vi "N4_201_write_P.vi"(0 "DriverConnect in":T1={"InterfaceType"=enum."VISA", "OpenedSession"="", "InterfaceSettings"={"Interface"=enum."RS232", "EOS 4 read"=enum."LF (\\n)", "EOS 4 write"=enum."LF (\\n)", "TMO, ms"=10000, "Sett"=variant(cluster{"Baud Rate":u32, "Data Bits":u16, "Parity":u16, "Stop Bits":u16, "Flow Control":u16, "Eho":bool} {"Baud Rate"=75, "Data Bits"=0, "Parity"=0, "Stop Bits"=0, "Flow Control"=0, "Eho"=FALSE})}}, 1 "P":T8, 2 "RangeIsChanged?":T6=TRUE, 3 "Command Time (s)":T7=1.0, 11 "error in":T9, 12 "Error Code":T11, 14 "Driver Name":T10) -> (4 "DriverConnect out":T1={"InterfaceType"=enum."VISA", "OpenedSession"="", "InterfaceSettings"={"Interface"=enum."RS232", "EOS 4 read"=enum."LF (\\n)", "EOS 4 write"=enum."LF (\\n)", "TMO, ms"=10000, "Sett"=variant(cluster{"Baud Rate":u32, "Data Bits":u16, "Parity":u16, "Stop Bits":u16, "Flow Control":u16, "Eho":bool} {"Baud Rate"=75, "Data Bits"=0, "Parity"=0, "Stop Bits"=0, "Flow Control"=0, "Eho"=FALSE})}}, 15 "error out":T9)   [LabVIEW 2018]
uses:
  MOKO_LabViewLibrary/MokoLowLevel/MokoLowLovelControl/MLLC_ErrorCode.ctl
  MOKO_LabViewLibrary/MokoLowLevel/MokoLowLovelControl/MLLC_DriverName.ctl
  MOKO_LabViewLibrary/MokoLowLevel/MokoLowLovelControl/MLLC_Error.ctl
  MOKO_LabViewLibrary/MokoLowLevel/MokoLowLovelControl/MLLC_Command.ctl
  MOKO_LabViewLibrary/MokoLowLevel/MokoLowLovelControl/MLLC_Delay.ctl
  MOKO_LabViewLibrary/MokoLowLevel/MokoLowLovelControl/MLLC_Boolean.ctl
  MOKO_LabViewLibrary/MokoLowLevel/MokoLowLovelControl/MLLC_DriverConnectCluster.ctl
  MOKO_LabViewLibrary/MokoLowLevel/MokoLowLovelControl/MLLC_InterfaceType.ctl
  MOKO_LabViewLibrary/MokoLowLevel/MokoLowLovelControl/MLLC_OpenedSession.ctl
  MOKO_LabViewLibrary/MokoLowLevel/MokoLowLovelControl/MLLC_InterfaceSettings.ctl
  MOKO_LabViewLibrary/MokoLowLevel/MokoLowLovelControl/MLLC_InterfaceKind.ctl
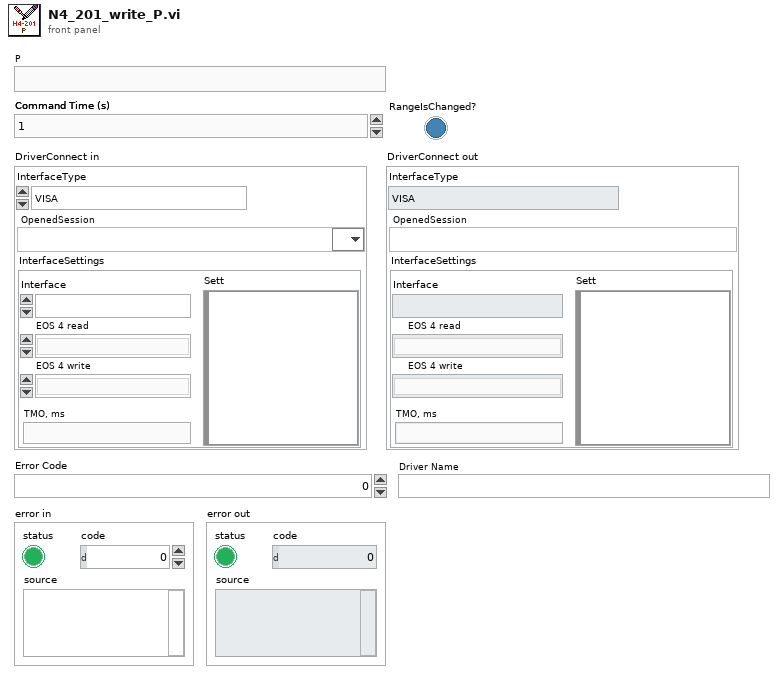
[diagram p1: front panel]
types:
  T1 = typedef "MLLC_DriverConnectCluster.ctl" = cluster{"InterfaceType":T2, "OpenedSession":T3, "InterfaceSettings":T4}
  T2 = typedef "MLLC_InterfaceType.ctl" = enum16{"VISA", "Prologix USB-GPIB"}
  T3 = typedef "MLLC_OpenedSession.ctl" = refnum<visa-resource-name>
  T4 = typedef "MLLC_InterfaceSettings.ctl" = cluster{"Interface":T5, "EOS 4 read":enum16{"Default (=EOS 4 write)", "CR (\\r)", "LF (\\n)", "None"}, "EOS 4 write":enum16{"CR+LF (\\r\\n)", "CR (\\r)", "LF (\\n)", "None"}, "TMO, ms":i32, "Sett":variant}
  T5 = typedef "MLLC_InterfaceKind.ctl" = enum16{"RS232", "GPIB", "USB", "Ethernet", "another"}
  T6 = typedef "MLLC_Boolean.ctl" = bool
  T7 = typedef "MLLC_Delay.ctl" = dbl
  T8 = typedef "MLLC_Command.ctl" = string
  T9 = typedef "MLLC_Error.ctl" = errorcluster
  T10 = typedef "MLLC_DriverName.ctl" = string
  T11 = typedef "MLLC_ErrorCode.ctl" = u32
  T12 = enum16{"Нет симуляции", "В ручную", "Игнорировать"}
  T13 = typedef "MLLC_Response.ctl" = string
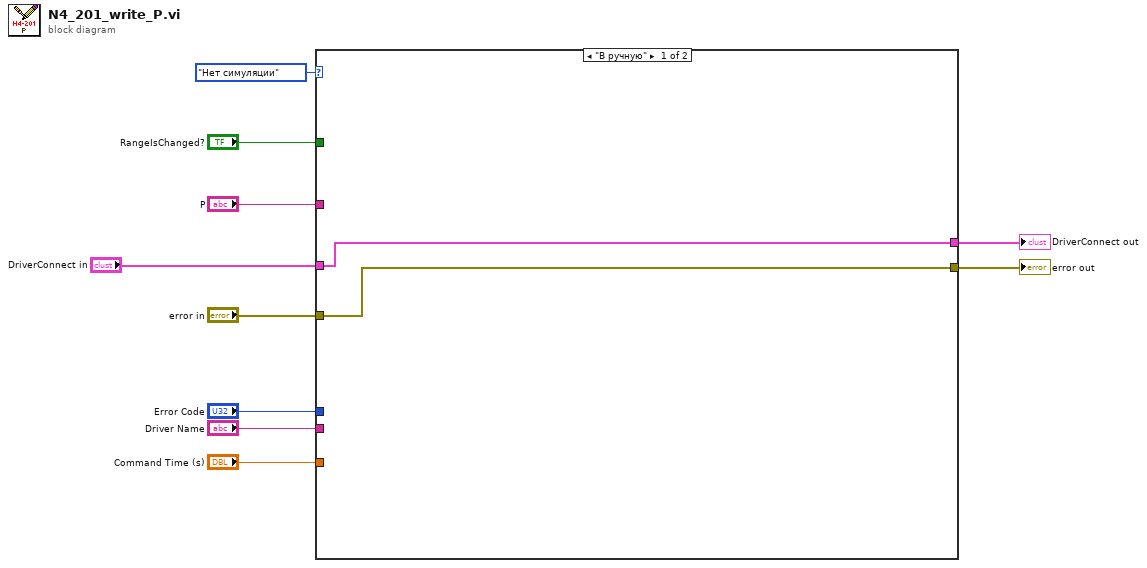
[diagram p0: block diagram]
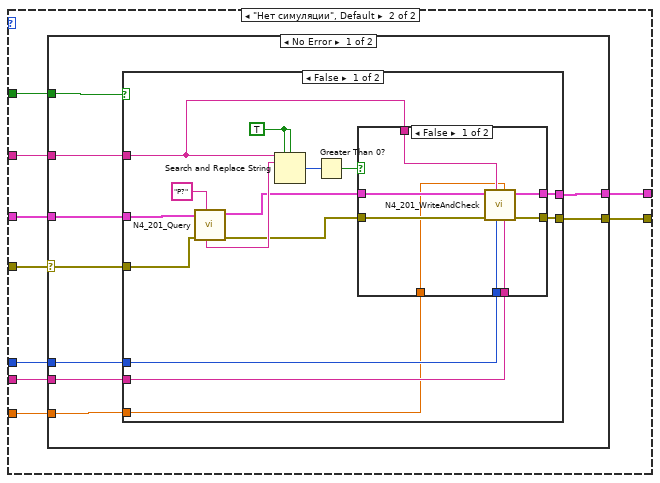
[diagram p2: hidden frame]
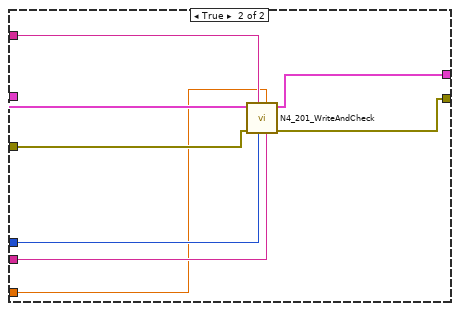
[diagram p4: hidden frame]
diagram:
  n1 = case shown="\"В ручную\"" T12."Нет симуляции" ("Simmulation") {
    tunnel: [w11 w21] -> w10
    tunnel: "Error Code" -> [_ w20]
    tunnel: "Driver Name" -> [_ w19]
    tunnel: "DriverConnect in" -> [w12 w18]
    tunnel: "error in" -> [w11 w17]
    tunnel: "P" -> [_ w16]
    tunnel: "Command Time (s)" -> [_ w15]
    tunnel: [w12 w14] -> w1
    tunnel: "RangeIsChanged?" -> [_ w13]
    frame "В ручную" {
    }
    frame "Нет симуляции", Default {
      n2 = case shown="No Error" w17 {
        selector: w17 -> [w25 w65]
        tunnel: [w27 w65] -> w21
        tunnel: [w28 w64] -> w14
        tunnel: w20 -> [w30 _]
        tunnel: w19 -> [w29 _]
        tunnel: w18 -> [w26 w64]
        tunnel: w16 -> [w24 _]
        tunnel: w15 -> [w22 _]
        tunnel: w13 -> [w23 _]
        frame No Error {
          n3 = case shown="False" w23 {
            tunnel: w30 -> [w36 w60]
            tunnel: w29 -> [w35 w59]
            tunnel: [w41 w62] -> w28
            tunnel: [w40 w61] -> w27
            tunnel: w22 -> [w34 w56]
            tunnel: w26 -> [w37 w58]
            tunnel: w25 -> [w38 w57]
            tunnel: w24 -> [w39 w63]
            frame False {
              w44 = TRUE ("replace all? (F)")
              n4 = call "N4_201_Query.vi"("Command"="P?" ("Error Query"), "error in"=w38, "DriverConnect in"=w37) -> ("error out"=w31:T9, "DriverConnect out"=w32:T1, "Response"=w33:T13)  [unwired: 6 in]
              n5 = Search and Replace String(replace all?=w44, case sensitive?=w44, input string=w39, search string=w33) -> (number of replacements=w43:i32)  [unwired: 4 in, 3 out]
              n6 = Greater Than 0?(x=w43) -> (x > 0?=w42:bool)
              n7 = case shown="False" w42 {
                tunnel: w36 -> [w53 _]
                tunnel: w35 -> [w52 _]
                tunnel: [w51 w55] -> w41
                tunnel: [w50 w54] -> w40
                tunnel: w34 -> [w46 _]
                tunnel: w39 -> [w49 _]
                tunnel: w32 -> [w47 w55]
                tunnel: w31 -> [w48 w54]
                frame False {
                  n8 = call "N4_201_WriteAndCheck.vi"("Driver Name"=w52, "Command Time (s)"=w46, "Error Code"=w53, "Command"=w49, "error in"=w48, "DriverConnect in"=w47) -> ("error out"=w50:T9, "DriverConnect out"=w51:T1)  [unwired: 4 in]
                }
                frame True {
                }
              }
            }
            frame True {
              n9 = call "N4_201_WriteAndCheck.vi"("Driver Name"=w59, "Command Time (s)"=w56, "Error Code"=w60, "Command"=w63, "error in"=w57, "DriverConnect in"=w58) -> ("error out"=w61:T9, "DriverConnect out"=w62:T1)  [unwired: 4 in]
            }
          }
        }
        frame Error {
        }
      }
    }
  }
  "error out" <- w10
  "DriverConnect out" <- w1
